vi "Boolean Debounce.vi"(7 "loops":i32, 8 "input":bool) -> (0 "output":bool)   [LabVIEW 2012, in "ProcessorHelperFunctions.lvlib"]
uses:
  ProcessorHelperFunctions.lvlib
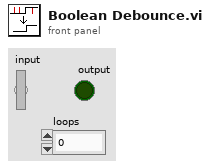
[diagram p1: front panel]
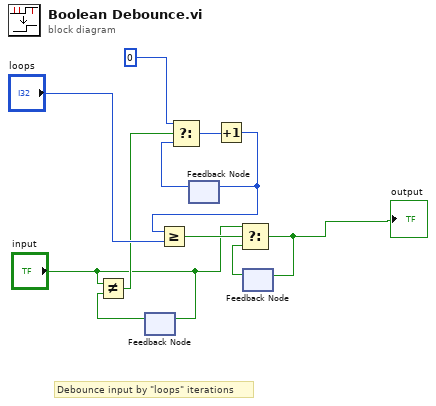
[diagram p0: block diagram]
diagram:
  # "Debounce input by \"loops\" iterations"
  n1 = feedback-in #1("input") -> ()
  n2 = feedback #1() -> (w8:bool)  [unwired: 1 in]
  n3 = Not Equal?(x="input", y=w8) -> (x != y?=w5:bool)
  n4 = feedback #2() -> (w10:i32)  [unwired: 1 in]
  n5 = Select(t=0, s=w5, f=w10) -> (s? t:f=w7:i32)
  n6 = Increment(x=w7) -> (x+1=w1:i32)
  n7 = Greater Or Equal?(x=w1, y="loops") -> (x >= y?=w9:bool)
  n8 = feedback-in #2(w1) -> ()
  n9 = feedback #3() -> (w4:bool)  [unwired: 1 in]
  n10 = Select(t="input", s=w9, f=w4) -> (s? t:f=w3:bool)
  "output" <- w3
  n11 = feedback-in #3(w3) -> ()
